vi "ExFileReadNDisplayRGBInteractiveTif.vi"() -> ()   [LabVIEW 2010]
panel:
  in  "Set values":bool
  in  "TIF output":path=path "C:/Program Files/SIToolKit/LabVIEW/Data Files/test"
  out "Blue Offset read":dbl format="%.2f"
  out "Green Offset read":dbl format="%.2f"
  out "Red Offset read":dbl format="%.2f"
  out "Blue Gain read":dbl format="%.2f"
  out "Green Gain read":dbl format="%.2f"
  out "Red Gain read":dbl format="%.2f"
  in  "Blue Offset":dbl format="%.2f"
  in  "Green Offset":dbl format="%.2f"
  in  "Red Offset":dbl format="%.2f"
  in  "Blue Gain":dbl=1.0 format="%.2f"
  in  "Red Gain":dbl=1.0 format="%.2f"
  in  "Green Gain":dbl=1.0 format="%.2f"
  in  "Bit shift":u16
  in  "Type of Bayer":u32=1 max=4 step=1
  in  "Full File Name":path=path "C:/Program Files/SIToolKit/LabVIEW/Data Files/Color.SPE"
  in  "?":bool
  in  "FileType":u32=67371008
  out "error out":errorcluster
  in  "error in (no error)":errorcluster
  # "ExReadFileNDisplayRGBInteractiveTif.vi\nThis example will read in a file of the selected data type and display as RGB frame. When finished viewing data, make sure to use the STOP button to close the display. This example allows the gain, bit shift and offsets to be \nset interactively."
  # "File Types:\nSPE = 67371008\nTIF   = 67174400\nPMI  = 67436544"
  # "Browse match pattern is set to *.spe.  Modify this if different file type is needed."
  # "Interactive section"
  # "This will properly close\nthe image and\ndeallocate memory."
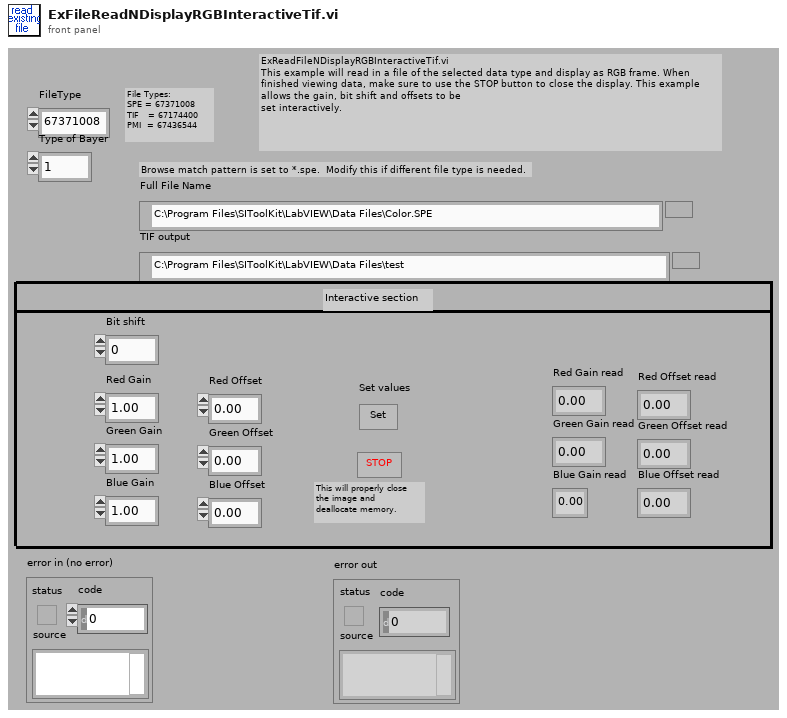
[diagram p1: front panel]
types:
  T1 = cluster{"Type of Bayer":u32, "Red Gain":dbl, "Green Gain":dbl, "Blue Gain":dbl, "Bit shift":u16, "Red Offset":dbl, "Green Offset":dbl, "Blue Offset":dbl}
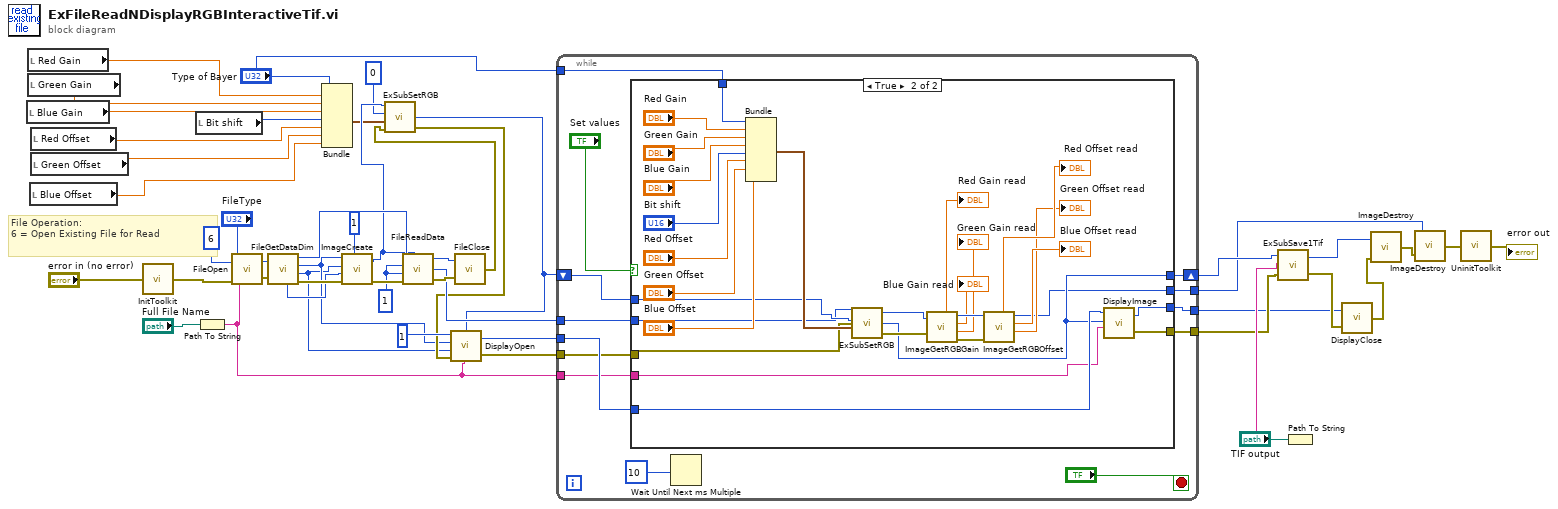
[diagram p0: block diagram]
diagram:
  w35 = 1
  # "File Operation:\n6 = Open Existing File for Read"
  n1 = local read "Blue Gain"() -> (w5:dbl)
  n2 = local read "Red Gain"() -> (w7:dbl)
  n3 = local read "Green Gain"() -> (w6:dbl)
  n4 = local read "Blue Offset"() -> (w2:dbl)
  n5 = local read "Red Offset"() -> (w4:dbl)
  n6 = local read "Green Offset"() -> (w3:dbl)
  n7 = call <userlib>:"InitToolkit.vi"("error in"="error in (no error)") -> ("error out"=w46:errorcluster)
  n8 = local read "Bit shift"() -> (w8:u16)
  n9 = Path To String(path="Full File Name") -> (string=w25:string)
  n10 = call <userlib>:"FileOpen.vi"("error in"=w46, "File Operations"=u32 6 ("File Operation"), "FileName"=w25, "File Type"="FileType") -> ("error out"=w44:errorcluster, "File Handle"=w43:u32)
  n11 = call <userlib>:"FileGetDataDim.vi"("File Handle"=w43, "error in"=w44) -> ("Data Type"=w12:u32, "File Handle"=w37:u32, "X dim"=w11:u32, "Y dim"=w10:u32, "error out"=w42:errorcluster)  [unwired: 1 out]
  n12 = Bundle("Type of Bayer"="Type of Bayer", "Red Gain"=w7, "Green Gain"=w6, "Blue Gain"=w5, "Bit shift"=w8, "Red Offset"=w4, "Green Offset"=w3, "Blue Offset"=w2) -> (w1:T1)  [unwired: 1 in]
  n13 = call <userlib>:"ImageCreate.vi"("X dimension"=w11, "Y dimension"=w10, "Data Type"=w12, "error in"=w42, "Number Of Frames"=1) -> ("Image Handle"=w16:u32, "error out"=w36:errorcluster)
  n14 = call <userlib>:"FileReadData.vi"("File Handle"=w37, "Start Frame"=w35, "End Frame"=w35, "error in"=w36, "Image Handle"=w16) -> ("File Handle"=w30:u32, "Image Handle"=w26:u32, "error out"=w29:errorcluster)
  n15 = call <userlib>:"FileClose.vi"("error in"=w29, "File Handle"=w30) -> ("error out"=w13:errorcluster)
  n16 = call "ExSubSetRGB.vi"("error in (no error)"=w13, "Adjustments"=w1, "RGB Handle"=0, "Image handle"=w16) -> ("error out"=w14:errorcluster, "RGB handle"=w9:u32)  [unwired: 1 out]
  n17 = call <userlib>:"DisplayOpen.vi"("Display Title"=w25, "Image Handle"=w9, "error in"=w14, "Display Height"=w10, "Display Width"=w11, "Display Type"=1) -> ("error out"=w27:errorcluster, "Display Handle"=w28:u32)
  n18 = while {
    tunnel: [w61] -> w23
    tunnel: w28 -> [w58]
    tunnel: w27 -> [w57]
    tunnel: w26 -> [w56]
    tunnel: w25 -> [w55]
    tunnel: [w54] -> w24
    tunnel: "Type of Bayer" -> [w52]
    shift-right: [w50] -> w19
    shift-left: w9 -> [w51]
    tunnel: [w49] -> w17
    stop <- "?" stop-if-true
    n19 = case shown="True" "Set values" {
      tunnel: [w63 w93] -> w61
      tunnel: w58 -> [w63 w84]
      tunnel: w57 -> [w62 w72]
      tunnel: w56 -> [w64 w68]
      tunnel: w55 -> [_ w83]
      tunnel: [w62 w82] -> w54
      tunnel: w52 -> [_ w78]
      tunnel: w51 -> [w65 w69]
      tunnel: [w65 w67] -> w50
      tunnel: [w64 w66] -> w49
      frame False {
      }
      frame True {
        n20 = Bundle("Type of Bayer"=w78, "Red Gain"="Red Gain", "Green Gain"="Green Gain", "Blue Gain"="Blue Gain", "Bit shift"="Bit shift", "Red Offset"="Red Offset", "Green Offset"="Green Offset", "Blue Offset"="Blue Offset") -> (w73:T1)  [unwired: 1 in]
        n21 = call "ExSubSetRGB.vi"("error in (no error)"=w72, "Adjustments"=w73, "RGB Handle"=w69, "Image handle"=w68) -> ("error out"=w71:errorcluster, "RGB handle"=w67:u32, "Image handle"=w70:u32)
        n22 = call <userlib>:"ImageGetRGBGain.vi"("Image Handle"=w70, "error in (no error)"=w71) -> ("Red"=→"Red Gain read":dbl, "Image Handle"=w91:u32, "Blue"=→"Blue Gain read":dbl, "Green"=→"Green Gain read":dbl, "error out"=w92:errorcluster)  [unwired: 1 out]
        n23 = call <userlib>:"ImageGetRGBOffset.vi"("Image Handle"=w91, "error in (no error)"=w92) -> ("Red"=→"Red Offset read":dbl, "Image Handle"=w66:u32, "Blue"=→"Blue Offset read":dbl, "Green"=→"Green Offset read":dbl)  [unwired: 2 out]
        n24 = call <userlib>:"DisplayImage.vi"("Title"=w83, "Image Handle"=w67, "Display Handle"=w84) -> ("error out"=w82:errorcluster, "Display Handle"=w93:u32)  [unwired: 1 in]
      }
    }
    n25 = Wait Until Next ms Multiple(millisecond multiple=10) -> ()  [unwired: 1 out]
  }
  n26 = Path To String(path="TIF output") -> (string=w31:string)
  n27 = call "ExSubSave1Tif.vi"("error in (no error)"=w24, "File name"=w31, "Image Handle"=w19) -> ("error out"=w33:errorcluster, "Image handle"=w18:u32)
  n28 = call <userlib>:"DisplayClose.vi"("error in"=w33, "Display Handle"=w23) -> ("error out"=w21:errorcluster)
  n29 = call <userlib>:"ImageDestroy.vi"("error in"=w21, "Data handle"=w18) -> ("error out"=w20:errorcluster)
  n30 = call <userlib>:"ImageDestroy.vi"("error in"=w20, "Data handle"=w17) -> ("error out"=w34:errorcluster)
  n31 = call <userlib>:"UninitToolkit.vi"("error in"=w34) -> ("error out"=→"error out":errorcluster)
